vi "Startup IO.vi"(8 "error in (no error)":errorcluster, 10 "Methods:Accessors:IO":refnum<class "IO.lvclass">, 11 "TopLevel in":refnum<class "TopLevel.lvclass">) -> (0 "error out":errorcluster)   [LabVIEW 2022 SP3, in "IO.lvclass"]
uses:
  IO.lvclass
  TopLevel/TopLevel.lvclass
  IO_Process.vi
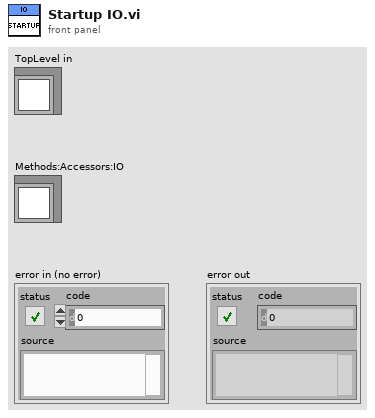
[diagram p1: front panel]
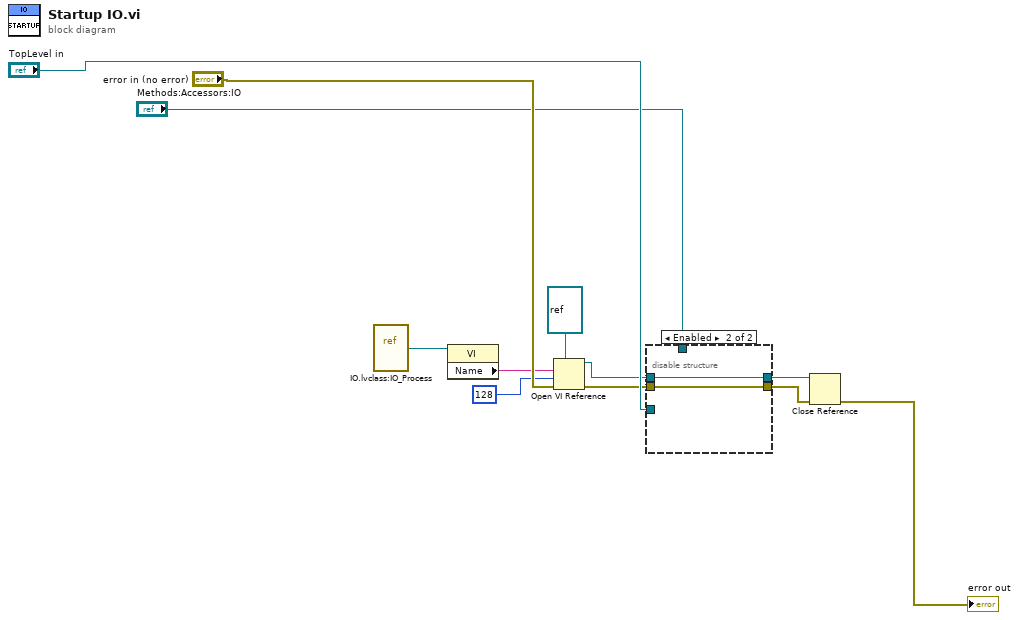
[diagram p0: block diagram]
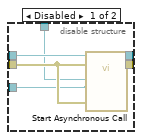
[diagram p2: hidden frame]
diagram:
  n1 = vi-ref "IO.lvclass:IO_Process.vi"() -> (w7:refnum<vi>)
  n2 = property class="VI"(reference=w7) -> ("Name"=w6:string)  [unwired: 1 in, 2 out]
  n3 = Open VI Reference(type specifier VI Refnum (for type only)=refnum<vi> refnum, vi path=w6, options=128, error in (no error)="error in (no error)") -> (vi reference=w4:refnum<vi>, error out=w3:errorcluster)  [unwired: 2 in]
  n4 = disable-structure shown="Enabled" {
    disable-tunnel: [w18 w19] -> w1
    disable-tunnel: [w17 w20] -> w2
    disable-tunnel: w3 -> [w16 w19]
    disable-tunnel: w4 -> [w15 w20]
    disable-tunnel: "Methods:Accessors:IO" -> [w14 _]
    disable-tunnel: "TopLevel in" -> [w13 _]
    frame Disabled {
      n5 = call-by-ref "Start Asynchronous Call"(reference=w15, error in=w16, "error in"=w16, "TopLevel"=w13, "IO in"=w14) -> (reference out=w17:refnum<vi>, error out=w18:errorcluster)  [unwired: 8 in, 1 out]
    }
    frame Enabled {
    }
  }
  n6 = Close Reference(reference=w2, error in (no error)=w1) -> (error out=→"error out":errorcluster)
